vi "readROIXML.vi"(8 "error in (no error)":errorcluster, 11 "ImageStreamViewer in":refnum<class "ImageStreamViewer.lvclass">) -> (0 "error out":errorcluster, 3 "ImageStreamViewer out":refnum<class "ImageStreamViewer.lvclass">)   [LabVIEW 2011, in "Views.lvlib" / "Camera.lvlib" / "ImageStreamViewer.lvclass"]
uses:
  ImageStreamViewer.lvclass
  ImageStreamViewer.lvclass/ImageStreamViewer.ctl
  Tools/NativeXML/NativeXML.lvclass
  Tools/Filing/FileSystem/FileSystem.lvclass
  Tools/Imaging.lvlib
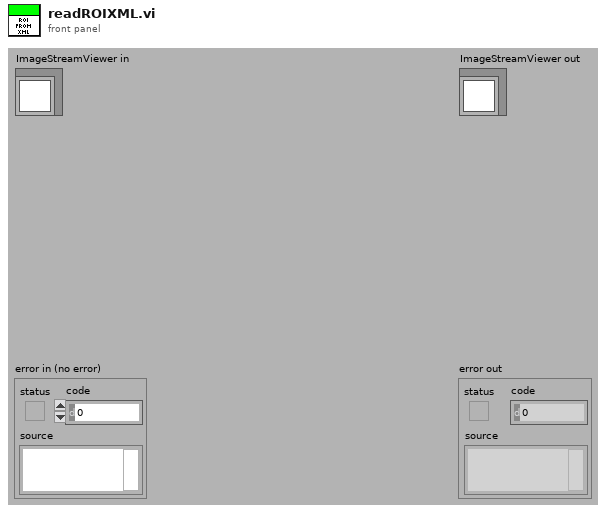
[diagram p1: front panel]
types:
  T1 = cluster{"Left":i32, "Top":i32, "Right":i32, "Bottom":i32}
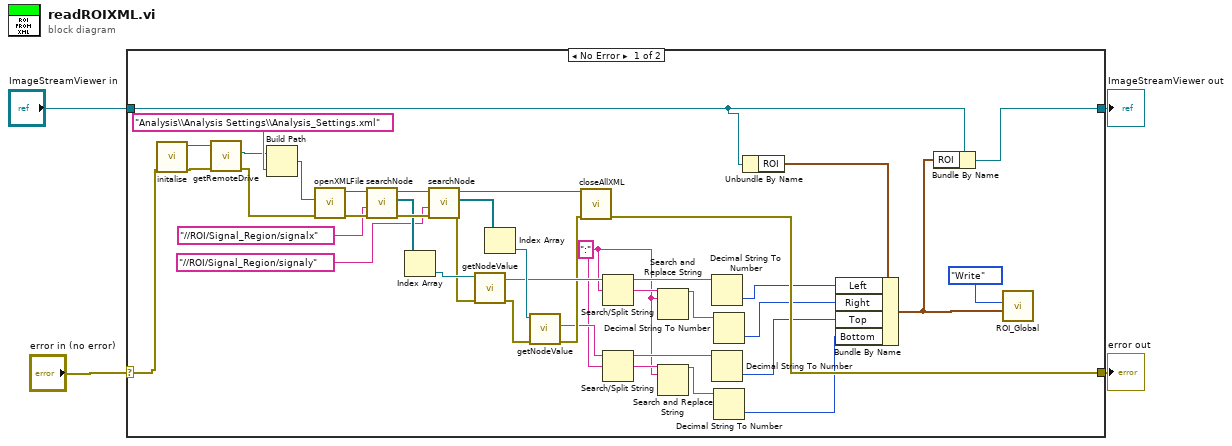
[diagram p0: block diagram]
diagram:
  n1 = case shown="No Error" "error in (no error)" {
    selector: "error in (no error)" -> [w27 w46]
    tunnel: [w26 w46] -> w3
    tunnel: [w10 w45] -> w1
    tunnel: "ImageStreamViewer in" -> [w11 w45]
    frame No Error {
      w9 = ":"
      n2 = call "initalise.vi"("error in (no error)"=w27) -> ("error out"=w33:errorcluster, "FileSystem out"=w32:refnum<class "FileSystem.lvclass">)  [unwired: 9 in]
      n3 = call "getRemoteDrive.vi"("error in (no error)"=w33, "FileSystem in"=w32) -> ("error out"=w28:errorcluster, "RemoteDrive"=w30:path)  [unwired: 7 in, 1 out]
      n4 = Build Path(base path=w30, name or relative path="Analysis\\Analysis Settings\\Analysis_Settings.xml") -> (appended path=w29:path)
      n5 = call "openXMLFile.vi"("error in (no error)"=w28, "Path"=w29) -> ("error out"=w43:errorcluster, "NativeXML out"=w44:refnum<class "NativeXML.lvclass">)  [unwired: 8 in]
      n6 = call "searchNode.vi"("error in (no error)"=w43, "searchXPath"="//ROI/Signal_Region/signalx", "NativeXML in"=w44) -> ("error out"=w41:errorcluster, "nodeArray"=w40:refnum<class "NativeXML.lvclass">[], "NativeXML out"=w42:refnum<class "NativeXML.lvclass">)  [unwired: 6 in]
      n7 = Index Array(array=w40) -> (element=w39:refnum<class "NativeXML.lvclass">)  [unwired: 1 in]
      n8 = call "searchNode.vi"("error in (no error)"=w41, "searchXPath"="//ROI/Signal_Region/signaly", "NativeXML in"=w42) -> ("error out"=w35:errorcluster, "nodeArray"=w38:refnum<class "NativeXML.lvclass">[], "NativeXML out"=w34:refnum<class "NativeXML.lvclass">)  [unwired: 6 in]
      n9 = call "getNodeValue.vi"("error in (no error)"=w35, "NativeXML in"=w39) -> ("error out"=w36:errorcluster, "Value"=w25:string)  [unwired: 7 in, 1 out]
      n10 = Index Array(array=w38) -> (element=w37:refnum<class "NativeXML.lvclass">)  [unwired: 1 in]
      n11 = call "getNodeValue.vi"("error in (no error)"=w36, "NativeXML in"=w37) -> ("error out"=w21:errorcluster, "Value"=w17:string)  [unwired: 7 in, 1 out]
      n12 = call "closeAllXML.vi"("error in (no error)"=w21, "NativeXML in"=w34) -> ("error out"=w26:errorcluster)  [unwired: 9 in]
      n13 = Search/Split String(string=w25, search string/char (-)=w9) -> (substring before match=w23:string, match + rest of string=w24:string)  [unwired: 1 in, 1 out]
      n14 = Search/Split String(string=w17, search string/char (-)=w9) -> (substring before match=w19:string, match + rest of string=w20:string)  [unwired: 1 in, 1 out]
      n15 = Search and Replace String(input string=w24, search string=w9) -> (result string=w22:string)  [unwired: 6 in, 3 out]
      n16 = Search and Replace String(input string=w20, search string=w9) -> (result string=w18:string)  [unwired: 6 in, 3 out]
      n17 = Decimal String To Number(string=w23) -> (number=w14:i32)  [unwired: 2 in, 1 out]
      n18 = Decimal String To Number(string=w19) -> (number=w13:i32)  [unwired: 2 in, 1 out]
      n19 = Decimal String To Number(string=w22) -> (number=w15:i32)  [unwired: 2 in, 1 out]
      n20 = Decimal String To Number(string=w18) -> (number=w12:i32)  [unwired: 2 in, 1 out]
      n21 = Unbundle By Name(w11) -> ("ROI"=w16:T1)
      n22 = Bundle By Name(cluster=w16, "Left"=w14, "Right"=w15, "Top"=w13, "Bottom"=w12) -> (w5:T1)
      n23 = Bundle By Name(cluster=w11, "ROI"=w5) -> (w10:refnum<class "ImageStreamViewer.lvclass">)
      n24 = call "ROI_Global.vi"("ROI"=w5, "Action"=enum16{"Write", "Read"}."Write") -> ()  [unwired: 9 in, 1 out]
    }
    frame Error {
    }
  }
  "error out" <- w3
  "ImageStreamViewer out" <- w1
